vi "DeleteBannedChars.vi"(8 "error in":errorcluster, 10 "string in":string, 11 "Log in":refnum<class "Log.lvclass">) -> (0 "error out":errorcluster, 2 "string out":string, 3 "Log out":refnum<class "Log.lvclass">)   [LabVIEW 2017, in "Reports.lvlib" / "Log.lvclass"]
doc: "This Method delete array of banned \nsymbols from input string"
uses:
  Log.lvclass
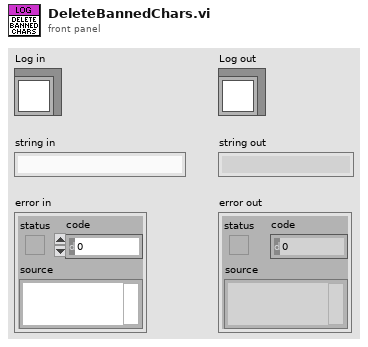
[diagram p1: front panel]
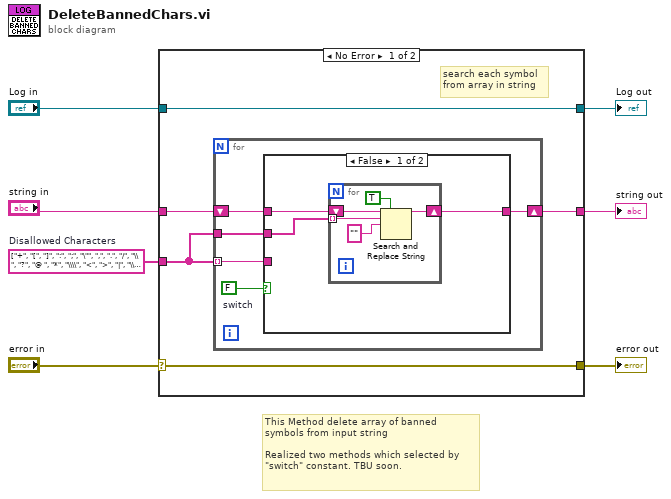
[diagram p0: block diagram]
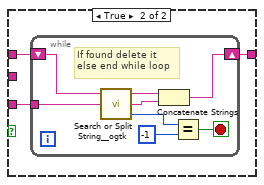
[diagram p2: hidden frame]
diagram:
  w2 = string[] ["+", "=", "[", "]", ":", ";", "\"", ",", ".", "/", "\\", "?", "@ ", "*", "\\\\", "<", ">", "|", "\\n", "\\r", "\\t"]  # Disallowed Characters
  # "This Method delete array of banned \nsymbols from input string\n\nRealized two methods which selected by\n\"switch\" constant. TBU soon."
  n1 = case shown="No Error" "error in" {
    selector: "error in" -> [w11 w38]
    tunnel: [w11 w38] -> w6
    tunnel: [w12 w37] -> w4
    tunnel: "Log in" -> [w12 w37]
    tunnel: [w10 _] -> w3
    tunnel: w2 -> [w8 _]
    tunnel: "string in" -> [w9 _]
    frame No Error {
      # "search each symbol\nfrom array in string"
      n2 = for {
        tunnel: w8 -> [w15] mode=indexing
        shift-right: [w16] -> w10
        shift-left: w9 -> [w17]
        tunnel: w8 -> [w13]
        w14 = FALSE  # switch
        n3 = case shown="False" w14 {
          tunnel: w17 -> [w20 w28]
          tunnel: [w19 w27] -> w16
          tunnel: w15 -> [_ w26]
          tunnel: w13 -> [w18 _]
          frame False {
            n4 = for {
              tunnel: w18 -> [w23] mode=indexing
              shift-right: [w21] -> w19
              shift-left: w20 -> [w24]
              n5 = Search and Replace String(replace all?=TRUE ("replace all? (F)"), input string=w24, search string=w23, replace string="" ("replace string (\"\")")) -> (result string=w21:string)  [unwired: 4 in, 3 out]
            }
          }
          frame True {
            n6 = while {
              shift-right: [w33] -> w27
              shift-left: w28 -> [w36]
              tunnel: w26 -> [w29]
              stop <- w30 stop-if-true
              # "If found delete it\nelse end while loop"
              n7 = call <userlib>:"Search or Split String__ogtk.vi"("search string/char (-)"=w29, "string"=w36) -> ("offset after match"=w32:i32, "substring after match"=w34:string, "substring before match"=w35:string)  [unwired: 1 in]
              n8 = Concatenate Strings(w35, w34) -> (w33:string)
              n9 = Equal?(x=w32, y=-1) -> (x = y?=w30:bool)
            }
          }
        }
      }
    }
    frame Error {
    }
  }
  "error out" <- w6
  "Log out" <- w4
  "string out" <- w3
